vi "Balance_200Hz.vi"() -> ()   [LabVIEW 2014]
uses:
  <vilib>/Platform/TimedLoop/XDataNode/timing_clust.ctl
  <vilib>/Platform/TimedLoop/XDataNode/nitl_modes.ctl
  <vilib>/Platform/TimedLoop/XDataNode/wakeup.ctl
  <vilib>/addons/control/pid/pid.llb/PID (DBL).vi
  <vilib>/platform/TimedLoop/XDataNode/XDataNode.xnode
  <vilib>/Platform/TimedLoop/XDataNode/XDNodeRunTimeDep.lvlib
  <userlib>/test_IMU/test_IMU.lvlib
  <vilib>/ptbypt/NI_PtbyPt.lvlib
  <vilib>/addons/control/pid/NI_PID_pid.lvlib
panel:
  out "Steering Adjustment":dbl format="%.2f"
  out "Gamma":dbl
  in  "Backward":bool
  in  "Forward":bool
  out "Iterations":i32
  out "Saturation counter":i32
  out "Controller Saturated":bool
  out "Theta Ref (Unsaturated)":dbl format="%0.2f"
  out "U  (Saturated)":sgl
  out "Phi Setpoint":dbl
  in  "stop":bool
  out "Mounted Angle":dbl
  out "Waveform Chart 3":T1(graph)
  out "Theta Ref (Saturated)":dbl format="%0.2f"
  out "Current Phi":dbl
  out "U (Unsaturated)":dbl format="%0.2f"
  out "Theta Error":dbl
  in  "Arm":bool
  out "Theta":dbl
  in  "Start Balance":bool
  out "Phi Error":dbl
  out "Encoder (ave)":dbl
  out "Theta Ref":cluster{"Filtered x":dbl, "val out":sgl}(graph)
  out "Output scale":sgl
  out "Waveform Chart":cluster{"Theta Setpoint":dbl, "val out":sgl}(graph)
  out "Theta Setpoint":dbl format="%0.2f"
  in  "Filter Time Constant":dbl=2.0 format="%#_13g"
  out "Current Theta":dbl
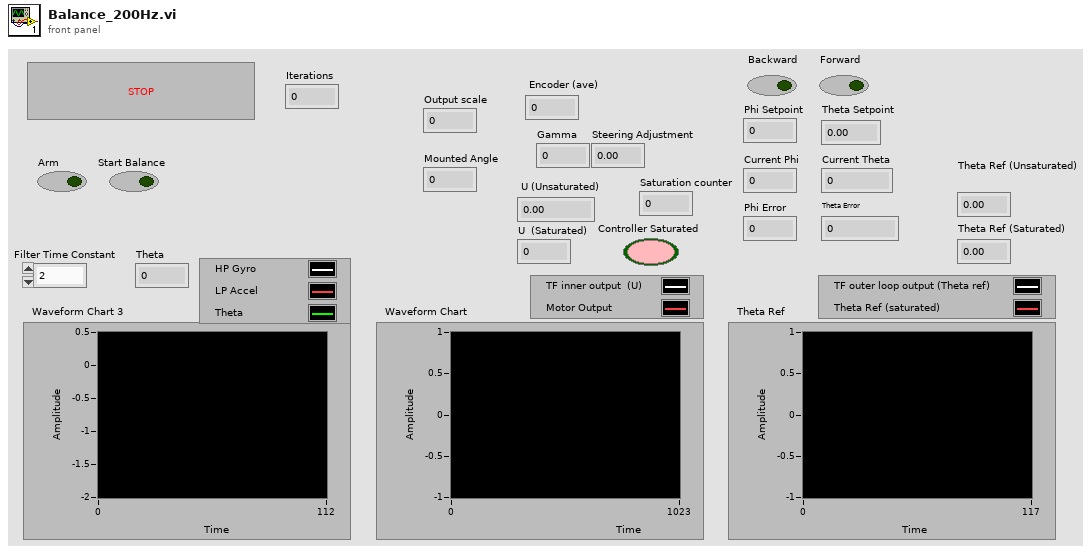
[diagram p1: front panel]
types:
  T1 = cluster{"HP Gyro ":dbl, "LP Accel":dbl, "Theta (rad)":dbl}
  T2 = cluster{"proportional gain (Kc)":dbl, "integral time (Ti, min)":dbl, "derivative time (Td, min)":dbl}
  T3 = cluster{"accel[0]":sgl, "accel[1]":sgl, "accel[2]":sgl, "gyro[0]":sgl, "gyro[1]":sgl, "gyro[2]":sgl, "mag[0]":sgl, "mag[1]":sgl, "mag[2]":sgl, "temp":sgl, "raw_gyro[0]":i16, "raw_gyro[1]":i16, "raw_gyro[2]":i16, "raw_accel[0]":i16, "raw_accel[1]":i16, "raw_accel[2]":i16, "accel_to_ms2":sgl, "gyro_to_degs":sgl, "dmp_quat[0]":sgl, "dmp_quat[1]":sgl, "dmp_quat[2]":sgl, "dmp_quat[3]":sgl, "dmp_TaitBryan[0]":sgl, "dmp_TaitBryan[1]":sgl, "dmp_TaitBryan[2]":sgl, "fused_quat[0]":sgl, "fused_quat[1]":sgl, "fused_quat[2]":sgl, "fused_quat[3]":sgl, "fused_TaitBryan[0]":sgl, "fused_TaitBryan[1]":sgl, "fused_TaitBryan[2]":sgl, "compass_heading":sgl}
  T4 = typedef "XDNodeRunTimeDep.lvlib/timing_clust.ctl" = cluster{"Expected End [f-1]":u64, "Actual End [f-1]":u64, "Finished Late? [f-1]":bool, "Expected End [i-1]":u64, "Actual End [i-1]":u64, "Finished Late? [i-1]":bool, "Expected Start [i]":u64, "Actual Start [i]":u64, "Expected Start [f]":u64, "Actual Start [f]":u64, "Source Name":string, "Structure Name":string, "Period":i64, "Deadline":i64, "Offset":i64, "Start":i64, "Priority":i32, "Timeout":i32, "Mode":T5, "Wakeup Reason":T6, "Error":errorcluster, "Source Type":string, "Secondary Source Type":string, "Global End Time":u64, "Global Start Time":u64, "Frame Duration":u64, "Iteration Duration":u64, "Assigned CPU":i32, "I/O Scan Engine Mode":u32}
  T5 = typedef "XDNodeRunTimeDep.lvlib/nitl_modes.ctl" = enum32{"No Change", "Process missed periods, maintain original phase", "Discard missed periods, maintain original phase", "Process missed periods, ignore original phase", "Discard missed periods, ignore original phase"}
  T6 = typedef "XDNodeRunTimeDep.lvlib/wakeup.ctl" = enum32{"Normal", "Aborted", "Asynchronous wakeup", "Timing source error", "Timed loop error", "Timeout"}
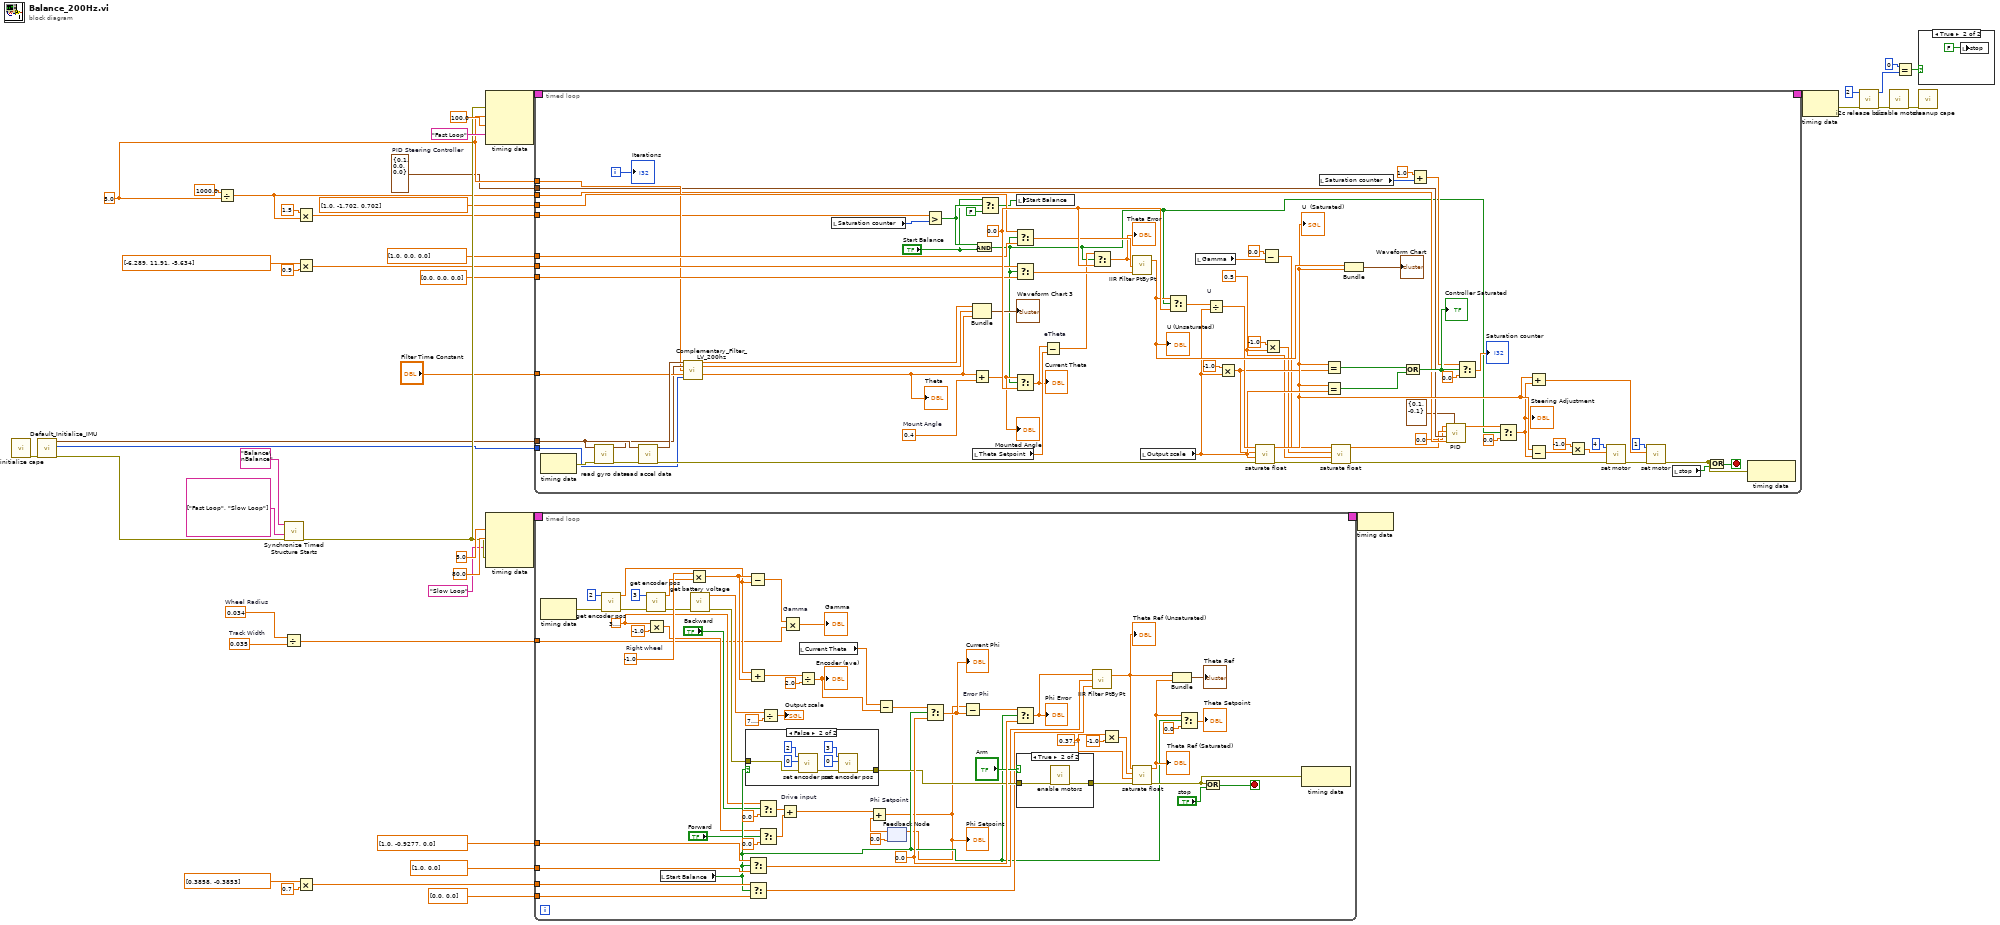
[diagram p0: block diagram]
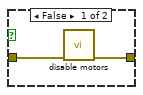
[diagram p3: hidden frame]
diagram:
  w2 = T2 {"proportional gain (Kc)"=0.1, "integral time (Ti, min)"=0.0, "derivative time (Td, min)"=0.0}  # PID Steering Controller
  w4 = 0.035  # Track Width
  w5 = 0.034  # Wheel Radius
  w11 = 5.0 ("Clock rate (ms) Inner Loop")
  n1 = call <userlib>:"initialize cape.vi"() -> ("error out"=w18:errorcluster)  [unwired: 10 in, 1 out]
  n2 = call <userlib>:"Default_Initialize_IMU.vi"("error in (no error)"=w18) -> ("error out"=w35:errorcluster, "Gyro FSR"=w33:i32, "data out"=w34:T3)  [unwired: 8 in]
  n3 = Divide(x=1000.0, y=w11) -> (x/y=w1:dbl)
  n4 = Divide(x=w5, y=w4) -> (x/y=w3:dbl)
  n5 = call <vilib>:"Synchronize Timed Structure Starts.vi"("error in (no error)"=w35, "timed structure names"=string[] ["Fast Loop", "Slow Loop"], "synchronization group name"="Balance\nBalance") -> ("error out"=w36:errorcluster)  [unwired: 7 in, 1 out]
  n6 = Multiply(x=1.5, y=w1) -> (x*y=w10:dbl)
  n7 = Multiply(x=dbl[] [-6.289, 11.91, -5.634] ("Denom Inner Loop"), y=0.9) -> (x*y=w24:dbl[])
  n8 = Multiply(x=dbl[] [0.3858, -0.3853] ("Denom Outer Loop"), y=0.7) -> (x*y=w20:dbl[])
  n9 = node-c288(w36, w11, 100.0 ("Priority Inner Loop"), "Fast Loop" ("Structure Name")) -> (w45:T4)
  n10 = node-c288(5.0 ("Clock rate (ms) Out Loop"), 80.0 ("Priority Outer Loop"), "Slow Loop" ("Structure Name"), w36) -> (w42:T4)
  n11 = timed-loop {
    timing: w45 -> [_]
    timing-out: [_] -> w44
    tunnel: w34 -> [w119]
    tunnel: w11 -> [w78]
    tunnel: "Filter Time Constant" -> [w116]
    tunnel: w33 -> [w88]
    tunnel: w24 -> [w102]
    tunnel: dbl[] [1.0, -1.702, 0.702] ("Num Inner Loop") -> [w105]
    tunnel: dbl[] [1.0, 0.0, 0.0] ("f") -> [w85]
    tunnel: dbl[] [0.0, 0.0, 0.0] ("f") -> [w84]
    tunnel: w10 -> [w66]
    tunnel: w2 -> [w64]
    tunnel: w1 -> [w63]
    i -> [w65]
    stop <- w86 stop-if-true
    w54 = 0.5
    w107 = 0.0 ("f")
    w118 = 0.4  # Mount Angle
    n12 = node-c288() -> (w120:errorcluster)  [unwired: 1 in]
    n13 = call <userlib>:"read gyro data.vi"("error in (no error)"=w120, "data"=w119) -> ("error out"=w121:errorcluster, "data out"=w93:T3)  [unwired: 7 in, 1 out]
    n14 = call <userlib>:"read accel data.vi"("error in (no error)"=w121, "data"=w119) -> ("error out"=w98:errorcluster, "data out"=w117:T3)  [unwired: 7 in, 1 out]
    n15 = call <userlib>:"Complementary_Filter_LV_200hz.vi"("Accel Data in"=w117, "Gyro Data in"=w93, "Dt( ms)"=w78, "Filter Time Constant"=w116, "gyro_fsr"=w88) -> ("HP Gyro"=w91:dbl, "LP Accel"=w92:dbl, "Theta (rad)"=w89:dbl)  [unwired: 7 in, 1 out]
    "Theta" <- w89
    n16 = local read "Saturation counter"() -> (w77:i32)
    n17 = Greater?(x=w66, y=w77) -> (0:w69:bool)
    n18 = Bundle("HP Gyro"=w91, "LP Accel"=w92, "Theta (rad)"=w89) -> (→"Waveform Chart 3":T1)  [unwired: 1 in]
    n19 = Add(x=w89, y=w118) -> (x+y=w97:dbl)
    "Mounted Angle" <- w97
    n20 = local read "Theta Setpoint"() -> (w95:dbl)
    n21 = And(x=w69, y="Start Balance") -> (x .and. y?=w46:bool)
    n22 = Select(t="Start Balance", s=w69, f=FALSE) -> (s? t:f=w70:bool)
    n23 = Select(t=w105, s=w46, f=w85) -> (s? t:f=w104:dbl[])
    n24 = Select(t=w102, s=w46, f=w84) -> (s? t:f=w101:dbl[])
    n25 = Select(t=w97, s=w46, f=w107) -> (s? t:f=w94:dbl)
    "Current Theta" <- w94
    n26 = local write "Start Balance"(w70) -> ()
    n27 = Subtract "eTheta"(x=w94, y=w95) -> (x-y=w99:dbl)
    n28 = Select(t=w99, s=w46, f=w107) -> (s? t:f=w100:dbl)
    "Theta Error" <- w100
    n29 = call <vilib>:"IIR Filter PtByPt.vi"("Forward Coefficients"=w101, "Reverse Coefficients"=w104, "x"=w100) -> ("Filtered x"=w103:dbl)  [unwired: 1 in, 1 out]
    "U (Unsaturated)" <- w103
    n30 = local read "Output scale"() -> (w83:sgl)
    n31 = Select(t=w103, s=w46, f=w107) -> (s? t:f=w108:dbl)
    n32 = local read "Gamma"() -> (w62:dbl)
    n33 = Divide "U"(x=w108, y=w83) -> (x/y=w96:dbl)
    n34 = Multiply(x=-1.0, y=w83) -> (x*y=w81:dbl)
    n35 = call <userlib>:"saturate float.vi"("error in (no error)"=w98, "max"=w83, "min"=w81, "val"=w96) -> ("error out"=w59:errorcluster, "val out"=w82:sgl)  [unwired: 5 in, 1 out]
    "U  (Saturated)" <- w82
    n36 = Subtract(x=0.0, y=w62) -> (x-y=w60:dbl)
    n37 = Multiply(x=-1.0, y=w54) -> (x*y=w53:dbl)
    n38 = local read "Saturation counter"() -> (w74:i32)
    n39 = Equal?(x=w82, y=w81) -> (x = y?=w79:bool)
    n40 = Equal?(x=w82, y=w83) -> (x = y?=w80:bool)
    n41 = call <userlib>:"saturate float.vi"("error in (no error)"=w59, "max"=w54, "min"=w53, "val"=w60) -> ("error out"=w58:errorcluster, "val out"=w57:sgl)  [unwired: 5 in, 1 out]
    n42 = Bundle("Filtered x"=w103, "val out"=w82) -> (→"Waveform Chart":cluster{"Filtered x":dbl, "val out":sgl})  [unwired: 1 in]
    n43 = Or(x=w79, y=w80) -> (x .or. y?=w76:bool)
    "Controller Saturated" <- w76
    n44 = Add(x=1.0 ("t"), y=w74) -> (x+y=w73:dbl)
    n45 = call-poly <vilib>:"PID.vi"("output range"=cluster{"output high":dbl, "output low":dbl} {"output high"=0.1, "output low"=-0.1}, "dt (s)"=w63, "PID gains"=w64, "process variable"=w57, "setpoint"=0.0) -> ("output"=w49:dbl)  [unwired: 5 in, 1 out]
    n46 = Select(t=w73, s=w76, f=0.0) -> (s? t:f=→"Saturation counter":dbl)
    n47 = Select(t=w49, s=w46, f=0.0) -> (s? t:f=w48:dbl)
    "Steering Adjustment" <- w48
    n48 = Add(x=w82, y=w48) -> (x+y=w51:dbl)
    n49 = Subtract(x=w82, y=w48) -> (x-y=w50:dbl)
    n50 = Multiply(x=-1.0, y=w50) -> (x*y=w110:dbl)
    n51 = call <userlib>:"set motor.vi"("error in (no error)"=w58, "duty"=w110, "motor"=4) -> ("error out"=w112:errorcluster)  [unwired: 7 in, 1 out]
    n52 = call <userlib>:"set motor.vi"("error in (no error)"=w112, "duty"=w51, "motor"=1) -> ("error out"=w111:errorcluster)  [unwired: 7 in, 1 out]
    n53 = local read "stop"() -> (w87:bool)
    n54 = Or(x=w111, y=w87) -> (x .or. y?=w86:bool)
    n55 = node-c288(w111) -> ()  [unwired: 1 out]
    "Iterations" <- w65
  }
  n56 = timed-loop {
    timing: w42 -> [_]
    timing-out: [_] -> w41
    tunnel: w20 -> [w159]
    tunnel: dbl[] [1.0, -0.9277, 0.0] ("Num Outer Loop") -> [w158]
    tunnel: dbl[] [1.0, 0.0] ("f") -> [w148]
    tunnel: dbl[] [0.0, 0.0] ("f") -> [w147]
    tunnel: w3 -> [w127]
    stop <- w152 stop-if-true
    w132 = 3.141592653589793
    w165 = 0.0 ("f")
    w172 = sgl 0.37 ("min")
    w177 = -1.0  # Right wheel
    n57 = node-c288() -> (w185:errorcluster)  [unwired: 1 in]
    n58 = call <userlib>:"get encoder pos.vi"("error in (no error)"=w185, "ch"=2) -> ("error out"=w182:errorcluster, "Output Angle"=w130:dbl)  [unwired: 8 in]
    n59 = call <userlib>:"get encoder pos.vi"("error in (no error)"=w182, "ch"=3) -> ("error out"=w176:errorcluster, "Output Angle"=w136:dbl)  [unwired: 8 in]
    n60 = Multiply(x=w132, y=-1.0) -> (x*y=w134:dbl)
    n61 = local read "Start Balance"() -> (w146:bool)
    n62 = Multiply(x=w177, y=w136) -> (x*y=w131:dbl)
    n63 = call <userlib>:"get battery voltage.vi"("error in (no error)"=w176) -> ("error out"=w167:errorcluster, "function return"=w175:sgl)  [unwired: 9 in]
    n64 = case shown="False" w146 {
      tunnel: w167 -> [w190 w192]
      tunnel: [w190 w191] -> w164
      frame True {
      }
      frame False {
        n65 = call <userlib>:"set encoder pos.vi"("error in (no error)"=w192, "value"=0, "ch"=2) -> ("error out"=w197:errorcluster)  [unwired: 7 in, 1 out]
        n66 = call <userlib>:"set encoder pos.vi"("error in (no error)"=w197, "value"=0, "ch"=3) -> ("error out"=w191:errorcluster)  [unwired: 7 in, 1 out]
      }
    }
    n67 = Subtract(x=w131, y=w130) -> (x-y=w129:dbl)
    n68 = Add(x=w130, y=w131) -> (x+y=w181:dbl)
    n69 = Select(t=w158, s=w146, f=w148) -> (s? t:f=w162:dbl[])
    n70 = Select(t=w159, s=w146, f=w147) -> (s? t:f=w160:dbl[])
    n71 = Select(t=w132, s="Backward", f=0.0) -> (s? t:f=w140:dbl)
    n72 = Select(t=w134, s="Forward", f=0.0) -> (s? t:f=w139:dbl)
    n73 = Divide(x=w175, y=sgl 7.4) -> (x/y=→"Output scale":sgl)
    n74 = Add "Drive input"(x=w140, y=w139) -> (x+y=w145:dbl)
    n75 = Multiply "Gamma"(x=w129, y=w127) -> (x*y=→"Gamma":dbl)
    n76 = Divide(x=w181, y=2.0) -> (x/y=w179:dbl)
    "Encoder (ave)" <- w179
    n77 = local read "Current Theta"() -> (w178:dbl)
    n78 = Subtract(x=w178, y=w179) -> (x-y=w166:dbl)
    n79 = feedback #1(0.0) -> (w138:dbl)
    n80 = Add "Phi Setpoint"(x=w145, y=w138) -> (x+y=w135:dbl)
    "Phi Setpoint" <- w135
    n81 = feedback-in #1(w135) -> ()
    n82 = Select(t=w166, s=w146, f=w165) -> (s? t:f=w161:dbl)
    "Current Phi" <- w161
    n83 = Subtract "Error Phi"(x=w135, y=w161) -> (x-y=w156:dbl)
    n84 = Select(t=w156, s=w146, f=w165) -> (s? t:f=w157:dbl)
    "Phi Error" <- w157
    n85 = case shown="True" "Arm" {
      tunnel: w164 -> [w187 w189]
      tunnel: [w186 w188] -> w155
      frame False {
        n86 = call <userlib>:"disable motors.vi"("error in (no error)"=w187) -> ("error out"=w186:errorcluster)  [unwired: 9 in, 1 out]
      }
      frame True {
        n87 = call <userlib>:"enable motors.vi"("error in (no error)"=w189) -> ("error out"=w188:errorcluster)  [unwired: 9 in, 1 out]
      }
    }
    n88 = call <vilib>:"IIR Filter PtByPt.vi"("Forward Coefficients"=w160, "Reverse Coefficients"=w162, "x"=w157) -> ("Filtered x"=w151:dbl)  [unwired: 1 in, 1 out]
    "Theta Ref (Unsaturated)" <- w151
    n89 = Multiply(x=w172, y=sgl -1.0) -> (x*y=w171:sgl)
    n90 = call <userlib>:"saturate float.vi"("error in (no error)"=w155, "max"=w172, "min"=w171, "val"=w151) -> ("error out"=w154:errorcluster, "val out"=w150:sgl)  [unwired: 5 in, 1 out]
    "Theta Ref (Saturated)" <- w150
    n91 = Bundle("Filtered x"=w151, "val out"=w150) -> (→"Theta Ref":cluster{"Filtered x":dbl, "val out":sgl})  [unwired: 1 in]
    n92 = Select(t=w150, s=w146, f=sgl 0.0) -> (s? t:f=→"Theta Setpoint":sgl)
    n93 = Or(x=w154, y="stop") -> (x .or. y?=w152:bool)
    n94 = node-c288(w154) -> ()  [unwired: 1 out]
  }
  n95 = node-c288(w41) -> ()
  n96 = node-c288(w44) -> (w29:errorcluster)
  n97 = call <userlib>:"i2c release bus.vi"("error in (no error)"=w29, "bus"=2) -> ("error out"=w27:errorcluster, "function return"=w8:i32)  [unwired: 8 in]
  n98 = call <userlib>:"disable motors.vi"("error in (no error)"=w27) -> ("error out"=w26:errorcluster)  [unwired: 9 in, 1 out]
  n99 = Equal?(x=0, y=w8) -> (x = y?=w9:bool)
  n100 = case shown="True" w9 {
    frame False {
    }
    frame True {
      n101 = local write "stop"(FALSE) -> ()
    }
  }
  n102 = call <userlib>:"cleanup cape.vi"("error in (no error)"=w26) -> ()  [unwired: 9 in, 2 out]
